vi "Test Noise Spectrum Level.vi"() -> ()   [LabVIEW 2015]
uses:
  Utility VIs/Math VIs/FFT x(t) to dB,Degrees (1D).vi
  Utility VIs/Math VIs/Linear to dB (scalar).vi
  <vilib>/Analysis/NI_AALBase.lvlib
panel:
  out "XY Graph":cluster{"Array":dbl[], "Array":dbl[]}[](graph)
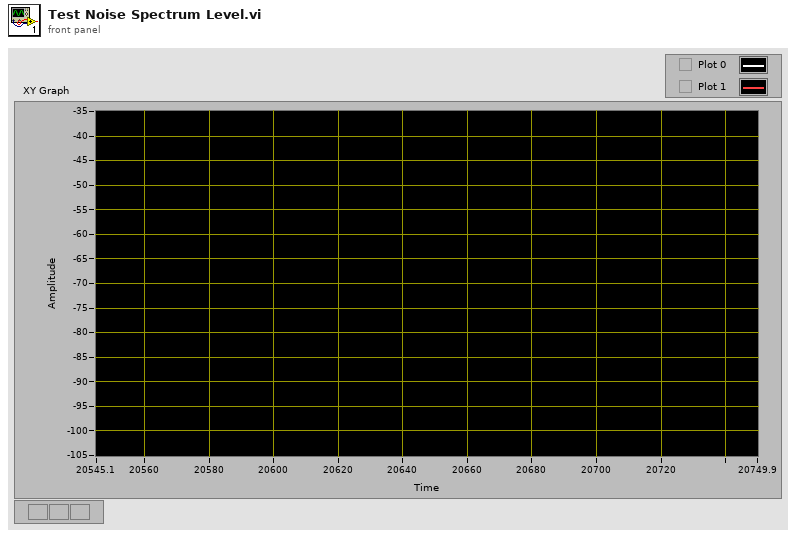
[diagram p1: front panel]
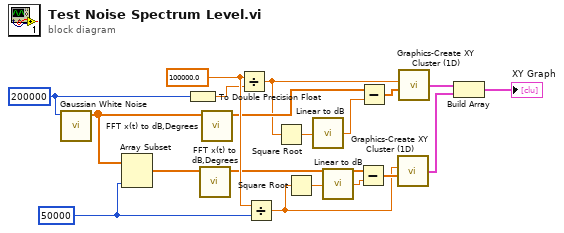
[diagram p0: block diagram]
diagram:
  w13 = 100000.0
  w14 = 50000
  w17 = 200000
  n1 = call <vilib>:"Gaussian White Noise.vi"("samples"=w17) -> ("Gaussian noise pattern"=w19:dbl[])  [unwired: 9 in, 1 out]
  n2 = Array Subset(array=w19, length=w14) -> (w18:dbl[])  [unwired: 1 in]
  n3 = To Double Precision Float(number=w17) -> (double precision float=w10:dbl)
  n4 = call-poly "FFT x(t) to dB,Degrees.vi"("X"=w18) -> ("+Freq. Mag of FFT (dB rms)"=w12:dbl[])  [unwired: 8 in, 2 out]
  n5 = call-poly "FFT x(t) to dB,Degrees.vi"("X"=w19) -> ("+Freq. Mag of FFT (dB rms)"=w9:dbl[])  [unwired: 8 in, 2 out]
  n6 = Divide(x=w13, y=w10) -> (x/y=w7:dbl)
  n7 = Divide(x=w13, y=w14) -> (x/y=w1:dbl)
  n8 = Square Root(x=w7) -> (sqrt(x)=w6:dbl)
  n9 = Square Root(x=w1) -> (sqrt(x)=w3:dbl)
  n10 = call-poly "Linear to dB.vi"("Linear"=w6) -> ("dB"=w5:dbl)
  n11 = call-poly "Linear to dB.vi"("Linear"=w3) -> ("dB"=w2:dbl)
  n12 = Subtract(x=w12, y=w2) -> (x-y=w4:dbl[])
  n13 = Subtract(x=w9, y=w5) -> (x-y=w8:dbl[])
  n14 = call "Graphics-Create XY Cluster (1D).vi"("Array"=w4, "dx"=w1) -> ("XY cluster"=w11:cluster{"Array":dbl[], "Array":dbl[]})  [unwired: 2 in]
  n15 = call "Graphics-Create XY Cluster (1D).vi"("Array"=w8, "dx"=w7) -> ("XY cluster"=w16:cluster{"Array":dbl[], "Array":dbl[]})  [unwired: 2 in]
  n16 = Build Array(w16, w11) -> (→"XY Graph":cluster{"Array":dbl[], "Array":dbl[]}[])
